vi "Create Plot Object.vi"(6 "Control Ref Queue":T1, 7 "Actual Transform In":T2, 8 "error in (no error)":errorcluster, 9 "Multiplot Representation In":T4, 10 "3D Mesh.lvclass in":refnum<class "3D Quiver.lvclass">, 11 "Plot Object In":refnum<vi>) -> (0 "error out":errorcluster, 1 "Multiplot Representation Out":T4, 2 "3D Mesh.lvclass out":refnum<class "3D Quiver.lvclass">, 3 "Plot Object Out":refnum<vi>, 5 "Actual Transform Out":T2)   [LabVIEW 2017, in "3D Quiver.lvclass"]
uses:
  <vilib>/Math Plots/3D Math Plots/3D Quiver/3D Quiver/3D Quiver.lvclass
  <vilib>/Math Plots/3D Math Plots/3D Plot/3D Plot/Typedef/Multiplot Representation.ctl
  <vilib>/Math Plots/3D Math Plots/3D Plot/3D Plot/Typedef/Plot Representation.ctl
  <vilib>/Math Plots/3D Math Plots/3D Plot/3D Plot/Typedef/Range Clusters.ctl
  <vilib>/Math Plots/3D Math Plots/3D Plot/3D Plot/Typedef/Mesh Data.ctl
  <vilib>/Math Plots/3D Math Plots/3D Plot/3D Plot/Typedef/Actual Transform.ctl
  <vilib>/Math Plots/3D Math Plots/3D Plot/Action String/3DMathPlot Ctrl Act Queue.ctl
  <vilib>/Math Plots/3D Math Plots/3D Plot/Action String/3DMathPlot Ctrl Act Cluster.ctl
  <vilib>/Math Plots/3D Math Plots/3D Plot/Action String/3DMathPlot State Class.ctl
  <vilib>/Math Plots/3D Math Plots/3D Quiver/3D Quiver/3D Quiver.lvclass/3D Quiver.ctl
  <vilib>/Math Plots/3D Math Plots/3D Plot/3D Plot/3D Plot.lvclass
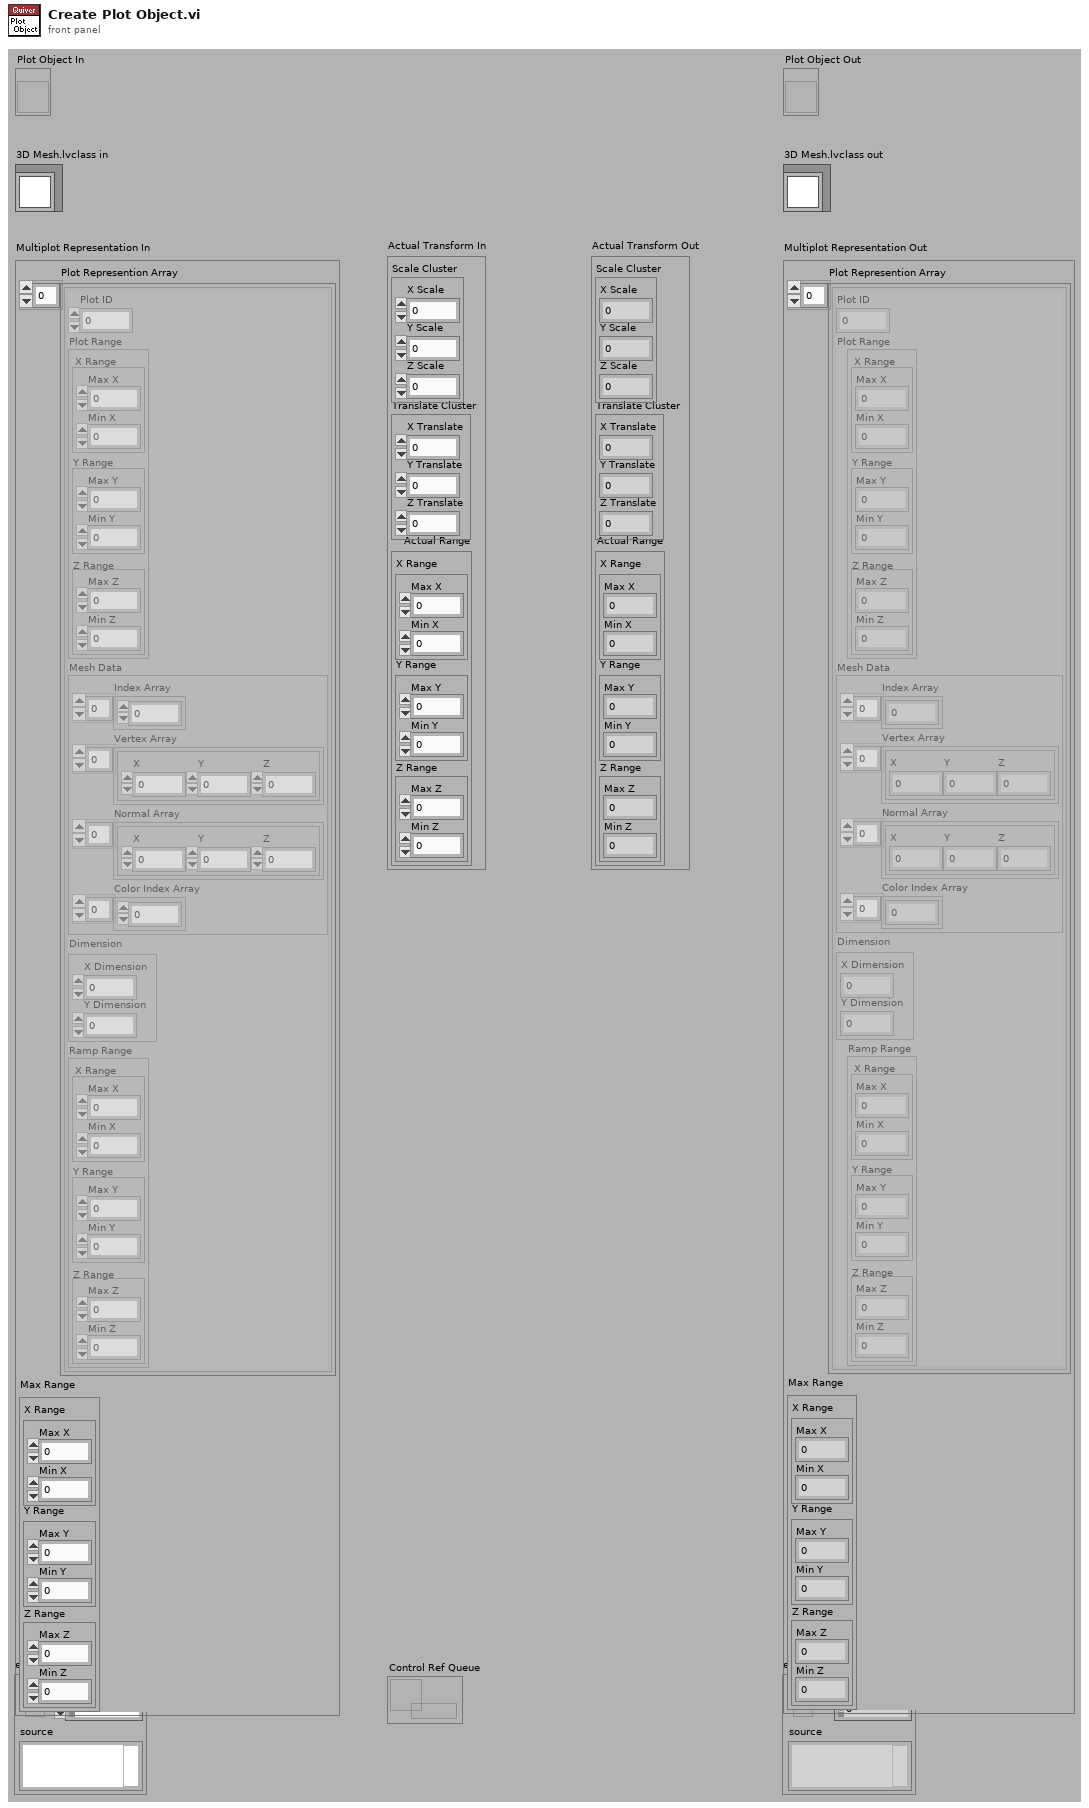
[diagram p1: front panel]
types:
  T1 = typedef "3DMathPlot Ctrl Act Queue.ctl" = refnum<queue>
  T2 = typedef "3D Plot.lvclass/Actual Transform.ctl" = cluster{"Scale Cluster":cluster{"X Scale":sgl, "Y Scale":sgl, "Z Scale":sgl}, "Translate Cluster":cluster{"X Translate":sgl, "Y Translate":sgl, "Z Translate":sgl}, "Actual Range":T3}
  T3 = typedef "3D Plot.lvclass/Range Clusters.ctl" = cluster{"X Range":cluster{"Max X":sgl, "Min X":sgl}, "Y Range":cluster{"Max Y":sgl, "Min Y":sgl}, "Z Range":cluster{"Max Z":sgl, "Min Z":sgl}}
  T4 = typedef "3D Plot.lvclass/Multiplot Representation.ctl" = cluster{"Plot Represention Array":T5[], "Max Range":T3}
  T5 = typedef "3D Plot.lvclass/Plot Representation.ctl" = cluster{"Plot ID":i32, "Plot Range":T3, "Mesh Data":T6, "Dimension":cluster{"X Dimension":i32, "Y Dimension":i32}, "Ramp Range":T3}
  T6 = typedef "3D Plot.lvclass/Mesh Data.ctl" = cluster{"Index Array":u32[], "Vertex Array":cluster{"X":sgl, "Y":sgl, "Z":sgl}[], "Normal Array":cluster{"X":sgl, "Y":sgl, "Z":sgl}[], "Color Index Array":i32[]}
  T7 = typedef "3D Quiver.lvclass/3D Quiver Property Array.ctl" = T8[]
  T8 = typedef "3D Quiver.lvclass/3D Quiver Property.ctl" = cluster{"General Property":cluster{"Plot Name":string, "Coordinate System":enum16{"Cartesian", "Cylindrical", "Spherical"}, "Opacity":sgl}, "Projection Property":cluster{"Draw XY":bool, "Draw YZ":bool, "Draw XZ":bool}, "Plot Property":cluster{"Line Style":T9, "Line Width":sgl, "Line Color":u32, "Antialiasing":bool, "Color Ramp Cluster":T10}, "Quiver Property":cluster{"Quvier Mode":enum16{"Quiver", "Quiver with surface"}, "Quiver Size":sgl, "Quiver Length":sgl}}
  T9 = typedef "3D Plot.lvclass/Line Type.ctl" = enum16{"None", "Solid", "Dash", "Dot", "Dash Dot"}
  T10 = typedef "3D Plot.lvclass/Color Ramp Cluster.ctl" = cluster{"Color Ramp Style":enum16{"None", "Shaded", "Color spectrum", "Grey scale", "Custom"}, "Color Ramp Array":u32[], "Color Ramp Index":i32[], "Interpolate?":bool, "Logarithm?":bool}
  T11 = enum16{"Points", "Lines", "Line Strip", "Line Loop", "Triangles", "Triangle Strip", "Triangle Fan", "Quads", "Quad Strip", "Polygon"}
  T12 = cluster{"Draw XY":bool, "Draw YZ":bool, "Draw XZ":bool}
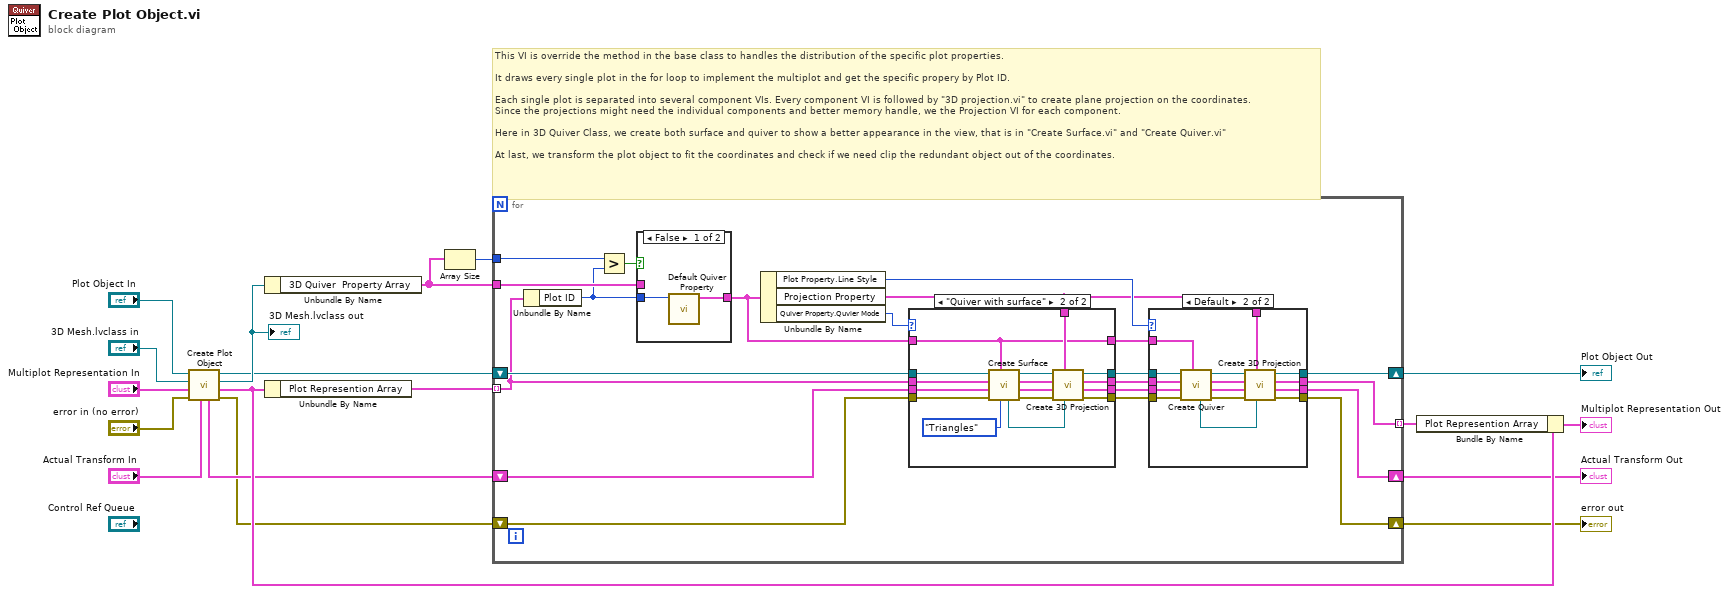
[diagram p0: block diagram]
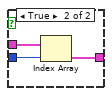
[diagram p2: hidden frame]
diagram:
  # "This VI is override the method in the base class to handles the distribution of the specific plot properties. \n\nIt draws every single plot in the for loop to implement the multiplot and get the specific propery by Plot ID.\n\nEach single plot is separated into several component VIs. Every component VI is followed by \"3D projection.vi\" to create plane projection on the coordinates. \nSince the projections might need the individual components and better memory handle, we the Projection VI for each component.\n\nHere in 3D Quiver Class, we create both surface and quiver to show a better appearance in the view, that is in \"Create Surface.vi\" and \"Create Quiver.vi\"\n\nAt last, we transform the plot object to fit the coordinates and check if we need clip the redundant object out of the coordinates."
  n1 = call-parent "Create Plot Object.vi"("Actual Transform In"="Actual Transform In", "error in (no error)"="error in (no error)", "Multiplot Representation In"="Multiplot Representation In", "3D Plot.lvclass in"="3D Mesh.lvclass in", "Plot Object In"="Plot Object In") -> ("error out"=w6:errorcluster, "Multiplot Representation Out"=w16:T4, "3D Plot.lvclass out"=w7:refnum<class "3D Quiver.lvclass">, "Plot Object Out"=w5:refnum<vi>, "Actual Transform Out"=w15:T2)  [unwired: 2 in]
  "3D Mesh.lvclass out" <- w7
  n2 = Unbundle By Name(w7) -> ("3D Quiver  Property Array"=w1:T7)
  n3 = Unbundle By Name(w16) -> ("Plot Represention Array"=w18:T5[])
  n4 = Array Size(array=w1) -> (size(s)=w2:i32)
  n5 = for {
    tunnel: [w36] -> w17 mode=indexing
    tunnel: w1 -> [w21]
    shift-right: [w34] -> w4
    shift-left: w5 -> [w39]
    shift-right: [w33] -> w8
    shift-left: w6 -> [w38]
    shift-right: [w32] -> w9
    shift-left: w15 -> [w35]
    tunnel: w18 -> [w31] mode=indexing
    tunnel: w2 -> [w20]
    n6 = Unbundle By Name(w31) -> ("Plot ID"=w19:i32)
    n7 = Greater?(x=w20, y=w19) -> (0:w23:bool)
    n8 = case shown="False" w23 {
      tunnel: w21 -> [_ w44]
      tunnel: [w40 w43] -> w22
      tunnel: w19 -> [w41 w42]
      frame False {
        n9 = call <vilib>:"Default Quiver Property.vi"("Plot ID"=w41) -> ("Default Property"=w40:T8)  [unwired: 10 out]
      }
      frame True {
        n10 = Index Array(array=w44, index=w42) -> (element=w43:T8)
      }
    }
    n11 = Unbundle By Name(w22) -> ("Plot Property.Line Style"=w25:T9, "Projection Property"=w24:T12, "Quiver Property.Quvier Mode"=w26:enum16{"Quiver", "Quiver with surface"})
    n12 = case shown="\"Quiver with surface\"" w26 {
      tunnel: w39 -> [w67 w82]
      tunnel: w38 -> [w64 w81]
      tunnel: [w66 w80] -> w37
      tunnel: w35 -> [w65 w79]
      tunnel: w31 -> [w66 w78]
      tunnel: [w67 w75] -> w30
      tunnel: [w65 w73] -> w29
      tunnel: [w64 w71] -> w28
      tunnel: w24 -> [_ w69]
      tunnel: w22 -> [w63 w68]
      tunnel: [w63 w68] -> w27
      frame "Quiver", Default {
      }
      frame "Quiver with surface" {
        n13 = call <vilib>:"Create Surface.vi"("Draw Mode"=T11."Triangles", "3D Quvier Property"=w68, "error in (no error)"=w81, "Actual Transform In"=w79, "Plot Representation In"=w78, "Plot Object In"=w82) -> ("error out"=w72:errorcluster, "Actual Transform Out"=w74:T2, "Plot Representation Out"=w80:T5, "Plot Object Out"=w76:refnum<vi>, "Surface Object Out"=w77:refnum<vi>)  [unwired: 1 in]
        n14 = call <vilib>:"Create 3D Projection.vi"("Sub Object In"=w77, "Projection Property"=w69, "error in (no error)"=w72, "Actual Transform In"=w74, "Plot Object In"=w76) -> ("error out"=w71:errorcluster, "Actual Transform Out"=w73:T2, "Plot Object Out"=w75:refnum<vi>)  [unwired: 1 in, 3 out]
      }
    }
    n15 = case shown="Default" w25 {
      tunnel: w37 -> [w47 w60]
      tunnel: [w47 w59] -> w36
      tunnel: [w48 w58] -> w34
      tunnel: [w45 w57] -> w33
      tunnel: [w46 w56] -> w32
      tunnel: w30 -> [w48 w53]
      tunnel: w29 -> [w46 w52]
      tunnel: w28 -> [w45 w51]
      tunnel: w27 -> [_ w50]
      tunnel: w24 -> [_ w49]
      frame "None" {
      }
      frame Default {
        n16 = call <vilib>:"Create Quiver.vi"("3D Quiver Property"=w50, "error in (no error)"=w51, "Actual Transform In"=w52, "Plot Representation In"=w60, "Plot Object In"=w53) -> ("error out"=w62:errorcluster, "Actual Transform Out"=w55:T2, "Plot Representation Out"=w59:T5, "Plot Object Out"=w61:refnum<vi>, "Quiver Object Out"=w54:refnum<vi>)  [unwired: 2 in]
        n17 = call <vilib>:"Create 3D Projection.vi"("Sub Object In"=w54, "Projection Property"=w49, "error in (no error)"=w62, "Actual Transform In"=w55, "Plot Object In"=w61) -> ("error out"=w57:errorcluster, "Actual Transform Out"=w56:T2, "Plot Object Out"=w58:refnum<vi>)  [unwired: 1 in, 3 out]
      }
    }
  }
  "error out" <- w8
  "Plot Object Out" <- w4
  "Actual Transform Out" <- w9
  n18 = Bundle By Name(cluster=w16, "Plot Represention Array"=w17) -> (→"Multiplot Representation Out":T4)
